vi "Write Laser Control.vi"(8 "error in (no error)":errorcluster, 10 "Laser Control":T1 {"Vrange" min=0 max=20}, 11 "Change PAS Laser Parameters in":refnum<class "Change PAS Laser Parameters.lvclass">) -> (0 "error out":errorcluster, 3 "Change PAS Laser Parameters out":refnum<class "Change PAS Laser Parameters.lvclass">)   [LabVIEW 2014, in "Change PAS Laser Parameters.lvclass"]
uses:
  Change PAS Laser Parameters.lvclass
  Change PAS Laser Parameters.lvclass/Change PAS Laser Parameters.ctl
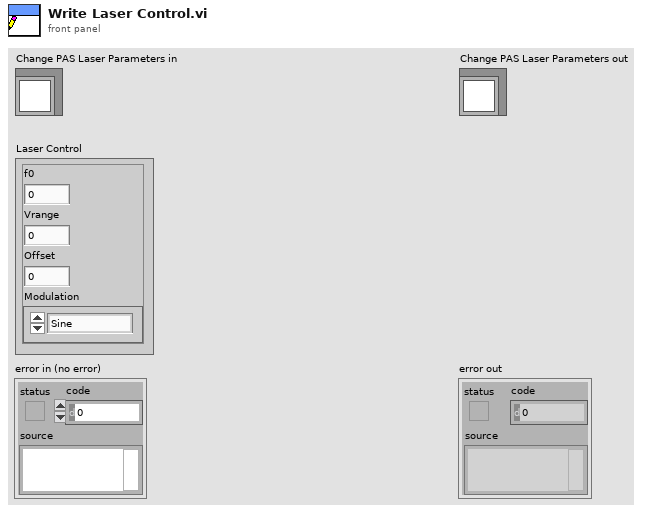
[diagram p1: front panel]
types:
  T1 = cluster{"f0":u16, "Vrange":sgl, "Offset":sgl, "Modulation":enum8{"Sine", "Square"}}
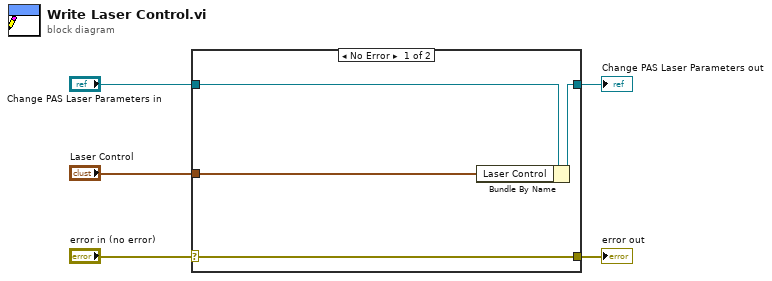
[diagram p0: block diagram]
diagram:
  n1 = case shown="No Error" "error in (no error)" {
    selector: "error in (no error)" -> [w9 w10]
    tunnel: [w9 w10] -> w4
    tunnel: [w7 w11] -> w2
    tunnel: "Change PAS Laser Parameters in" -> [w8 w11]
    tunnel: "Laser Control" -> [w6 _]
    frame No Error {
      n2 = Bundle By Name(cluster=w8, "Laser Control"=w6) -> (w7:refnum<class "Change PAS Laser Parameters.lvclass">)
    }
    frame Error {
    }
  }
  "error out" <- w4
  "Change PAS Laser Parameters out" <- w2
